vi "encoder_test_3mode.vi"() -> ()   [LabVIEW 2014]
uses:
  <vilib>/rvi/FXPMathLib/FxpSinAndCos/subVIs/nifxpmath_SinAndCos_SimConfig.ctl
  <vilib>/rvi/Emulation/niFpgaGetClockAttributes.vi
  <vilib>/rvi/Emulation/niFpgaSctlEmulationGetInTimedLoop.vi
  <vilib>/rvi/Emulation/niFpgaEmulationReportErrorSimple.vi
  <vilib>/rvi/eio/common/nirviEmuTemplateMethod_errors.vi
  <vilib>/rvi/Emulation/niFpgaProcessEmulError.vi
  <vilib>/rvi/Emulation/niFpgaCriticalErrorInLSC.vi
  <vilib>/rvi/FXPMathLib/FxpSinAndCos/simVIs/DllFxpSinAndCosTemp_sub.vi
  <vilib>/rvi/interface/RandomDataEmulation/nirviRandomDataMultiElementFPGAFIFO.vi
  <instcachedir>/0/nirviRandomDataMultiElementFPGAFIFO_AD0CFC12EF974623A9C2E4184BC062B2.lvgen/nirviRandomDataMultiElementFPGAFIFO_AD0CFC12EF974623A9C2E4184BC062B2_023.vi
  <vilib>/rvi/interface/RandomDataEmulation/niFpgaRandomDataHandleErrors.vi
  <vilib>/eio/EIONode/EIONode.xnode
  <vilib>/rvi/FXPMathLib/FxpMul/XNode/nifxpmath_Multiplier.xnode
  <vilib>/rvi/FXPMathLib/FxpSinAndCos/XNode/nifxpmath_SinAndCos.xnode
  <vilib>/rvi/Analysis/measure/butterworth/XNode/niFpgaButterworthFilter.xnode
  <vilib>/rvi/FXPMathLib/FxpSub/XNode/nifxpmath_Sub.xnode
  <vilib>/rvi/FXPMathLib/FxpAdd/XNode/nifxpmath_Add.xnode
  <vilib>/rvi/DataTransferAndStorage/Container/XNode/niFpgaContainer.xnode
  <vilib>/rvi/interface/RandomDataEmulation/nirviRandomDataFpgaMultiElementTemplate.vi
  <vilib>/rvi/FXPMathLib/sim/FxpSim.dll
panel:
  out "omega (M_avg)":fxp<+/-,64,35>
  out "D_d (M_avg)":fxp<+/-,64,32>
  in  "D_d_M_avg_Tc (uSec)":u32
  out "omega (M)":fxp<+/-,64,30>
  out "D_d (M)":fxp<+/-,64,27>
  in  "D_d_M_Tc (uSec)":u32 format="%#_6f"
  out "D_d (T)":fxp<+/-,46,10>
  out "omega(T)":fxp<+/-,20,9>
  in  "Velocity Estimation":i16(ring) items=["M_avg method", "M method", "T method"]
  out "Dr_ramp":fxp<+/-,64,30>
  out "Dr_slope":fxp<+/-,33,17>
  in  "Dr_time":fxp<+/-,16,11>
  out "Dr_sin":fxp<+/-,28,11>
  out "Dr_sin_d":fxp<+/-,64,16>
  out "Dr_sin_dd":fxp<+/-,64,25>
  out "Sin omega":fxp<+/-,41,8>
  in  "Sin offset":fxp<+/-,27,10>
  in  "Sin magnitude":fxp<+/-,11,8>
  in  "Sin wave frequency (Hz)":fxp<+/-,21,5>
  out "Time now (s)":fxp<+,52,14>
  out "Dr":fxp<+/-,64,31>
  in  "Dr_end":fxp<+/-,16,11>
  in  "Command type":i16(ring) items=["Step", "Ramp", "Sine"]
  out "D_i":fxp<+/-,34,18>
  in  "D_tolorence":fxp<+/-,14,3>
  in  "Ki":fxp<+/-,20,6>
  out "D_error":fxp<+/-,24,11>
  in  "Direction":bool
  out "Fmr_PD":fxp<+/-,64,31>
  in  "Kd":fxp<+/-,20,8>
  in  "Kp":fxp<+/-,20,12>
  in  "scaled coefficients_D_dd":i32[](array[numeric])=[780119100, 146811362]
  out "D_dd":fxp<+/-,36,29>
  in  "Ini coe.":bool
  out "va":fxp<+/-,38,8>
  out "vb":fxp<+/-,38,8>
  in  "stop motor":bool
  out "vq_F":fxp<+/-,20,5> format="%.57g"
  out "vd_F":fxp<+/-,20,5>
  out "D_d (mm/s)":fxp<+/-,32,12>
  out "mt":u32
  out "omega (rad/s)":fxp<+/-,32,18>
  in  "mt0":u32
  out "D(mm)":fxp<+/-,22,7>
  out "rad(NrTheta)":fxp<+/-,33,18>
  out "Encoder Position":i32
  in  "Encoder Reset":bool
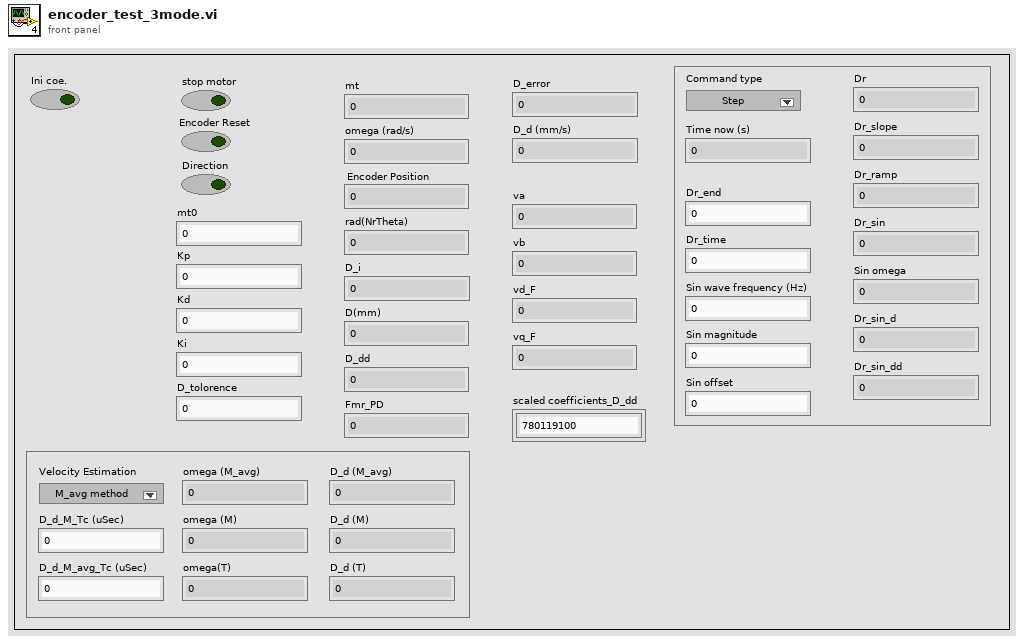
[diagram p1: front panel]
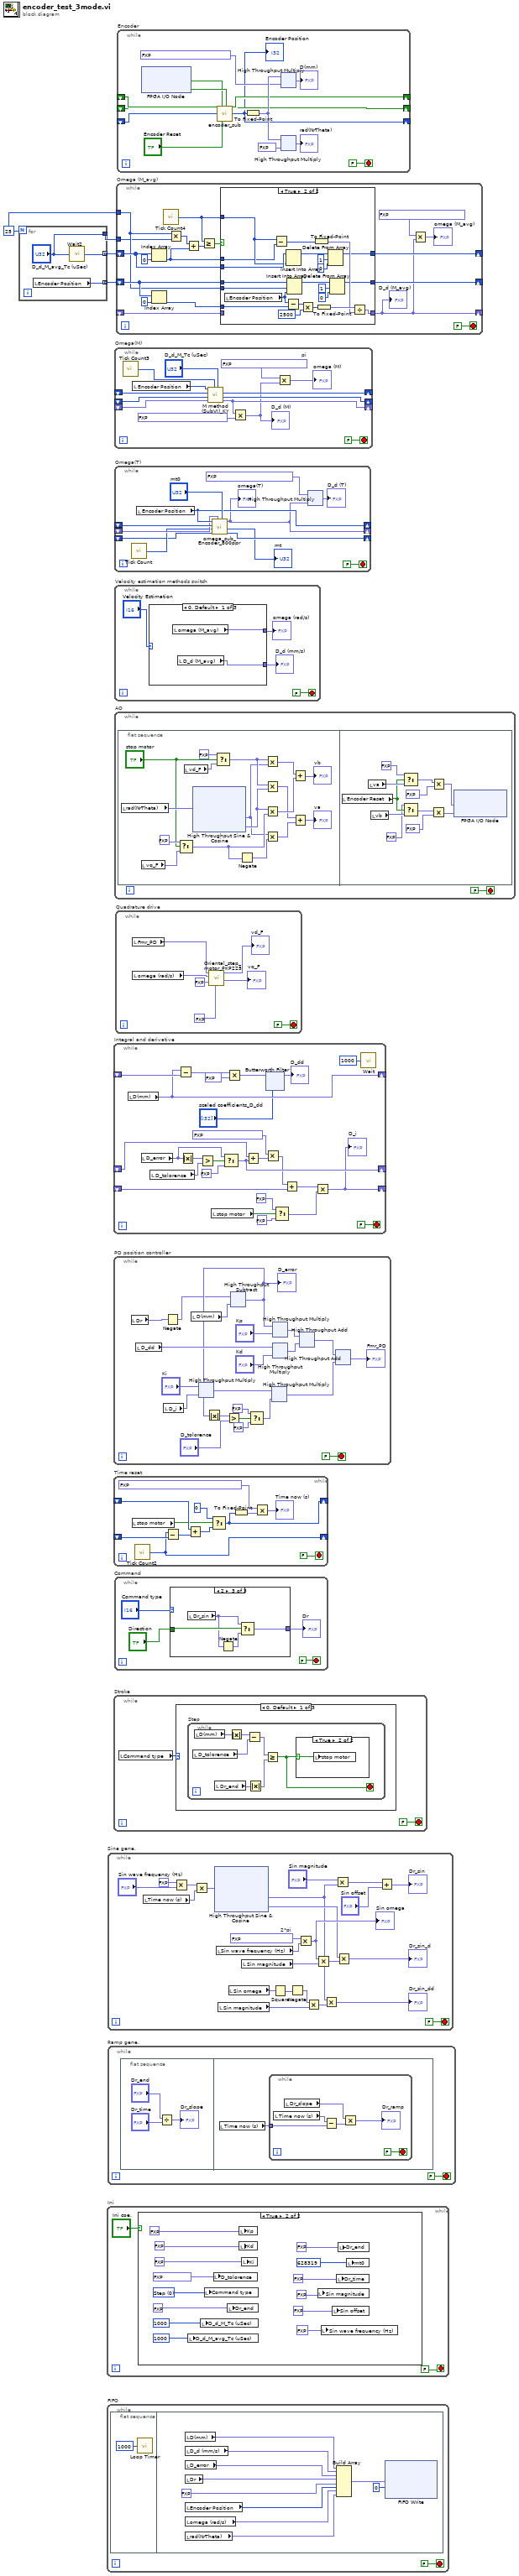
[diagram p0: block diagram]
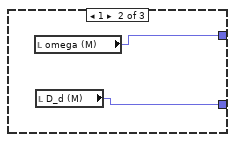
[diagram p3: hidden frame]
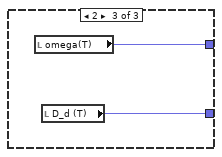
[diagram p4: hidden frame]
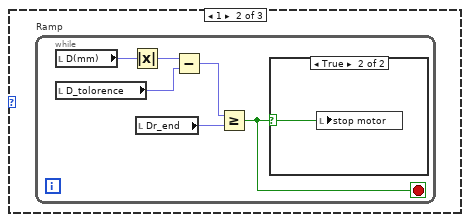
[diagram p6: hidden frame]
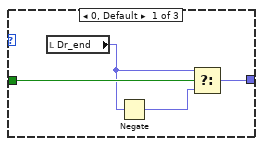
[diagram p9: hidden frame]
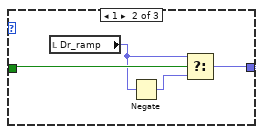
[diagram p10: hidden frame]
diagram:
  w4 = 25
  n1 = for {
    N: w4 -> [_]
    tunnel: ["D_d_M_avg_Tc (uSec)"] -> w1
    tunnel: [w6] -> w3 mode=indexing
    tunnel: [w5] -> w2 mode=indexing
    n2 = local read "Encoder Position"() -> (w5:i32)
    n3 = call "Wait2"("Count(uSec)"="D_d_M_avg_Tc (uSec)") -> ("Tick Count(uSec)"=w6:u32)
  }
  n4 = while "Ini" {
    stop <- FALSE stop-if-true
    n5 = case shown="True" "Ini coe." {
      frame False {
      }
      frame True {
        w17 = i16 0 items=["Step", "Ramp", "Sine"] ("Command type")
        n6 = local write "D_d_M_avg_Tc (uSec)"(u32 1000 ("D_d_M_avg_Tc (uSec)")) -> ()
        n7 = local write "D_d_M_Tc (uSec)"(u32 1000 ("D_d_M_Tc (uSec)")) -> ()
        n8 = local write "Command type"(w17) -> ()
        n9 = local write "D_tolorence"(fxp<+/-,14,3> 0.009765625 ("D_tolorence")) -> ()
        n10 = local write "Dr_end"(fxp<+/-,16,11> 20.0 ("Dr_end")) -> ()
        n11 = local write "Kp"(fxp<+/-,20,12> 10.0 ("Kp")) -> ()
        n12 = local write "Kd"(fxp<+/-,20,8> 2.0 ("Kd")) -> ()
        n13 = local write "Ki"(fxp<+/-,20,6> 8.0 ("D_i")) -> ()
        n14 = local write "Sin magnitude"(fxp<+/-,11,8> 20.0 ("Sin magnitude")) -> ()
        n15 = local write "Sin wave frequency (Hz)"(fxp<+/-,21,5> 0.5 ("Sin wave frequency (Hz)")) -> ()
        n16 = local write "Sin offset"(fxp<+/-,27,10> 0.0 ("Sin offset")) -> ()
        n17 = local write "Dr_time"(fxp<+/-,16,11> 5.0 ("Dr_time")) -> ()
        n18 = local write "Dr_end"(fxp<+/-,11,7> 20.0 ("Fmr")) -> ()
        n19 = local write "mt0"(u32 628319 ("mt0")) -> ()
      }
    }
  }
  n20 = while "FIFO" {
    stop <- FALSE stop-if-true
    n21 = flat-sequence {
      frame #0 {
        n22 = call "Loop Timer"("Count(uSec)"=u32 1000) -> ()  [unwired: 1 out]
      }
      frame #1 {
        n23 = local read "D(mm)"() -> (w33:fxp<+/-,22,7>)
        n24 = local read "D_d (mm/s)"() -> (w32:fxp<+/-,32,12>)
        n25 = local read "D_error"() -> (w31:fxp<+/-,24,11>)
        n26 = local read "Dr"() -> (w30:fxp<+/-,64,31>)
        n27 = local read "Encoder Position"() -> (w29:i32)
        n28 = local read "omega (rad/s)"() -> (w28:fxp<+/-,32,18>)
        n29 = local read "rad(NrTheta)"() -> (w27:fxp<+/-,33,18>)
        n30 = Build Array(w33, w32, w31, w30, fxp<+/-,64,32> 0.0 ("element"), w29, w28, w27) -> (w34:fxp<+/-,64,32>[])
        n31 = xnode ("FIFO Write")("Element"=w34, "Timeout"=0) -> ()  [unwired: 1 in, 2 out]
      }
    }
  }
  n32 = while "Sine gene." {
    stop <- FALSE stop-if-true
    w53 = fxp<+,20,3> 6.2831878662109375  # 2*pi
    n33 = local read "Time now (s)"() -> (w56:fxp<+,52,14>)
    n34 = Multiply(x=fxp<+,1,2> 2.0, y="Sin wave frequency (Hz)") -> (x*y=w57:fxp<+/-,21,6>)
    n35 = Multiply(x=w57, y=w56) -> (x*y=w37:fxp<+/-,64,20>)
    n36 = xnode "High Throughput Sine & Cosine"("x (pi)"=w37) -> ("sin(x)"=w41:fxp<+/-,16,2>, "cos(x)"=w48:fxp<+/-,16,2>)
    n37 = local read "Sin wave frequency (Hz)"() -> (w52:fxp<+/-,21,5>)
    n38 = local read "Sin magnitude"() -> (w43:fxp<+/-,11,8>)
    n39 = local read "Sin omega"() -> (w44:fxp<+/-,41,8>)
    n40 = local read "Sin magnitude"() -> (w47:fxp<+/-,11,8>)
    n41 = Square(x=w44) -> (x^2=w45:fxp<+,64,14>)
    n42 = Negate(x=w45) -> (-x=w42:fxp<+/-,64,15>)
    n43 = Multiply(x=w53, y=w52) -> (x*y=w49:fxp<+/-,41,8>)
    "Sin omega" <- w49
    n44 = Multiply(x=w42, y=w43) -> (x*y=w46:fxp<+/-,64,23>)
    n45 = Multiply(x=w49, y=w47) -> (x*y=w54:fxp<+/-,51,15>)
    n46 = Multiply(x=w41, y=w46) -> (x*y=→"Dr_sin_dd":fxp<+/-,64,25>)
    n47 = Multiply(x="Sin magnitude", y=w41) -> (x*y=w55:fxp<+/-,27,10>)
    n48 = Multiply(x=w48, y=w54) -> (x*y=→"Dr_sin_d":fxp<+/-,64,16>)
    n49 = Add(x=w55, y="Sin offset") -> (x+y=→"Dr_sin":fxp<+/-,28,11>)
  }
  n50 = while "Ramp gene." {
    stop <- FALSE stop-if-true
    n51 = flat-sequence {
      frame #0 {
        n52 = Divide(x="Dr_end", y="Dr_time") -> (x/y=→"Dr_slope":fxp<+/-,33,17>)
      }
      frame #1 {
        n53 = local read "Time now (s)"() -> (w94:fxp<+,52,14>)
        n54 = while {
          tunnel: w94 -> [w100]
          stop <- FALSE stop-if-true
          n55 = local read "Time now (s)"() -> (w97:fxp<+,52,14>)
          n56 = local read "Dr_slope"() -> (w98:fxp<+/-,33,17>)
          n57 = Subtract(x=w97, y=w100) -> (x-y=w99:fxp<+/-,53,15>)
          n58 = Multiply(x=w98, y=w99) -> (x*y=→"Dr_ramp":fxp<+/-,64,30>)
        }
      }
    }
  }
  n59 = while "Integral and derivative" {
    shift-right: [w121] -> _
    shift-left: _ -> [w125]
    shift-right: [w111] -> _
    shift-left: _ -> [w112]
    shift-right: [w101] -> _
    shift-left: _ -> [w105]
    stop <- FALSE stop-if-true
    n60 = local read "D(mm)"() -> (w121:fxp<+/-,22,7>)
    n61 = local read "D_error"() -> (w113:fxp<+/-,24,11>)
    n62 = local read "D_tolorence"() -> (w116:fxp<+/-,14,3>)
    n63 = Subtract(x=w121, y=w125) -> (x-y=w124:fxp<+/-,23,8>)
    n64 = Absolute Value(x=w113) -> (abs(x)=w117:fxp<+,24,11>)
    n65 = Greater?(x=w117, y=w116) -> (0:w115:bool)
    n66 = local read "stop motor"() -> (w108:bool)
    n67 = Select(t=w113, s=w115, f=fxp<+,24,11> 0.0) -> (s? t:f=w111:fxp<+/-,25,12>)
    n68 = Multiply(x=w124, y=fxp<+/-,33,13> 1000.0) -> (x*y=w122:fxp<+/-,55,20>)
    n69 = Add(x=w112, y=w111) -> (x+y=w110:fxp<+/-,26,13>)
    n70 = Multiply(x=fxp<+/-,30,12> 0.000499725341796875, y=w110) -> (x*y=w104:fxp<+/-,55,24>)
    n71 = xnode "Butterworth Filter"("input data"=w122, "scaled coefficients"="scaled coefficients_D_dd") -> ("output data"=→"D_dd":fxp<+/-,36,24>)  [unwired: 1 in]
    n72 = Select(t=fxp<+,1,1> 0.0, s=w108, f=fxp<+,1,1> 1.0) -> (s? t:f=w102:fxp<+,1,1>)
    n73 = Add(x=w104, y=w105) -> (x+y=w103:fxp<+/-,32,16>)
    n74 = Multiply(x=w103, y=w102) -> (x*y=w101:fxp<+/-,32,16>)
    "D_i" <- w101
    n75 = call "Wait"("Count(uSec)"=u32 1000) -> ()  [unwired: 1 out]
  }
  n76 = while "PD position controller" {
    stop <- FALSE stop-if-true
    n77 = local read "Dr"() -> (w136:fxp<+/-,64,31>)
    n78 = local read "D_dd"() -> (w152:fxp<+/-,36,29>)
    n79 = local read "D_i"() -> (w147:fxp<+/-,34,18>)
    n80 = Negate(x=w136) -> (-x=w135:fxp<+/-,64,32>)
    n81 = local read "D(mm)"() -> (w156:fxp<+/-,22,7>)
    n82 = xnode ("High Throughput Multiply")("x"="Ki", "y"=w147) -> ("x*y"=w141:fxp<+/-,54,24>)
    n83 = xnode "High Throughput Subtract"("x"=w135, "y"=w156) -> ("x-y"=w145:fxp<+/-,64,33>)
    "D_error" <- w145
    n84 = Absolute Value(x=w145) -> (abs(x)=w146:fxp<+,64,33>)
    n85 = Greater?(x=w146, y="D_tolorence") -> (0:w144:bool)
    n86 = Select(t=fxp<+,10,2> 1.0, s=w144, f=fxp<+,10,2> 0.0) -> (s? t:f=w140:fxp<+,10,2>)
    n87 = xnode ("High Throughput Multiply")("x"=w141, "y"=w140) -> ("x*y"=w137:fxp<+/-,64,26>)
    n88 = xnode ("High Throughput Multiply")("x"=w145, "y"="Kp") -> ("x*y"=w154:fxp<+/-,64,45>)
    n89 = xnode ("High Throughput Multiply")("x"=w152, "y"="Kd") -> ("x*y"=w153:fxp<+/-,56,37>)
    n90 = xnode ("High Throughput Add")("x"=w154, "y"=w153) -> ("x+y"=w138:fxp<+/-,64,46>)
    n91 = xnode ("High Throughput Add")("x"=w138, "y"=w137) -> ("x+y"=→"Fmr_PD":fxp<+/-,64,47>)
  }
  n92 = while "Time reset" {
    shift-right: [w160] -> _
    shift-left: _ -> [w167]
    shift-right: [w162] -> _
    shift-left: _ -> [w163]
    stop <- FALSE stop-if-true
    n93 = local read "stop motor"() -> (w165:bool)
    n94 = call "Tick Count2"() -> ("Tick Count(uSec)"=w162:u32)
    n95 = Subtract(x=w162, y=w163) -> (x-y=w168:u32)
    n96 = Add(x=w167, y=w168) -> (x+y=w166:u32)
    n97 = Select(t=u32 0, s=w165, f=w166) -> (s? t:f=w160:u32)
    n98 = To Fixed-Point(number=w160) -> (fixed-point=w159:fxp<+,32,32>)  [unwired: 1 in]
    n99 = Multiply(x=fxp<+,20,-18> 1.0000003385357559e-06, y=w159) -> (x*y=→"Time now (s)":fxp<+,52,14>)
  }
  n100 = while "Stroke" {
    stop <- FALSE stop-if-true
    n101 = local read "Command type"() -> (w170:i16)
    n102 = case shown="0, Default" w170 {
      frame 0, Default {
        n103 = while "Step" {
          stop <- w171 stop-if-true
          n104 = local read "D_tolorence"() -> (w173:fxp<+/-,14,3>)
          n105 = local read "D(mm)"() -> (w175:fxp<+/-,22,7>)
          n106 = local read "Dr_end"() -> (w177:fxp<+/-,16,11>)
          n107 = Absolute Value(x=w175) -> (abs(x)=w174:fxp<+,22,7>)
          n108 = Subtract(x=w174, y=w173) -> (x-y=w172:fxp<+/-,23,8>)
          n109 = Absolute Value(x=w177) -> (abs(x)=w176:fxp<+,16,11>)
          n110 = Greater Or Equal?(x=w172, y=w176) -> (x >= y?=w171:bool)
          n111 = case shown="True" w171 {
            selector: w171 -> [_ w178]
            frame False {
            }
            frame True {
              n112 = local write "stop motor"(w178) -> ()
            }
          }
        }
      }
      frame 1 {
        n113 = while "Ramp" {
          stop <- w179 stop-if-true
          n114 = local read "D(mm)"() -> (w181:fxp<+/-,22,7>)
          n115 = local read "D_tolorence"() -> (w183:fxp<+/-,14,3>)
          n116 = Absolute Value(x=w181) -> (abs(x)=w182:fxp<+,22,7>)
          n117 = local read "Dr_end"() -> (w180:fxp<+/-,16,11>)
          n118 = Subtract(x=w182, y=w183) -> (x-y=w184:fxp<+/-,23,8>)
          n119 = Greater Or Equal?(x=w184, y=w180) -> (x >= y?=w179:bool)
          n120 = case shown="True" w179 {
            selector: w179 -> [_ w185]
            frame False {
            }
            frame True {
              n121 = local write "stop motor"(w185) -> ()
            }
          }
        }
      }
      frame 2 {
      }
    }
  }
  n122 = while "Command" {
    stop <- FALSE stop-if-true
    n123 = case shown="2" "Command type" {
      tunnel: [w190 w194 w198] -> w188
      tunnel: "Direction" -> [w193 w197 w201]
      frame 0, Default {
        n124 = local read "Dr_end"() -> (w192:fxp<+/-,16,11>)
        n125 = Negate(x=w192) -> (-x=w191:fxp<+/-,17,12>)
        n126 = Select(t=w192, s=w193, f=w191) -> (s? t:f=w190:fxp<+/-,17,12>)
      }
      frame 1 {
        n127 = local read "Dr_ramp"() -> (w195:fxp<+/-,64,30>)
        n128 = Negate(x=w195) -> (-x=w196:fxp<+/-,64,31>)
        n129 = Select(t=w195, s=w197, f=w196) -> (s? t:f=w194:fxp<+/-,64,31>)
      }
      frame 2 {
        n130 = local read "Dr_sin"() -> (w199:fxp<+/-,28,11>)
        n131 = Negate(x=w199) -> (-x=w200:fxp<+/-,27,10>)
        n132 = Select(t=w199, s=w201, f=w200) -> (s? t:f=w198:fxp<+/-,28,11>)
      }
    }
    "Dr" <- w188
  }
  n133 = while "Omega(M)" {
    shift-right: [w213] -> _
    shift-left: _ -> [w214]
    shift-right: [w209] -> _
    shift-left: _ -> [w210]
    shift-right: [w207] -> _
    shift-left: _ -> [w208]
    stop <- FALSE stop-if-true
    w204 = fxp<+/-,27,3> 3.1415926218032837  # pi
    n134 = call "Tick Count3"() -> ("Tick Count(mSec)"=w212:u32)
    n135 = local read "Encoder Position"() -> (w215:i32)
    n136 = call "M method (SubVI)_KY.vi"("Tc (mSec)"="D_d_M_Tc (uSec)", "Tick Count (mSec)"=w212, "Encoder velocity_pre (pulse/s)"=w208, "Shift Register in 2"=w210, "Shift Register in 1"=w214, "Encoder pulses"=w215) -> ("Encoder velocity (pulse/s)"=w207:fxp<+/-,64,32>, "Shift Register out 2"=w209:i32, "Shift Register out 1"=w213:u32)  [unwired: 3 in]
    n137 = Multiply(x=w207, y=fxp<+/-,20,-5> 0.002499997615814209) -> (x*y=w205:fxp<+/-,64,27>)
    "D_d (M)" <- w205
    n138 = Multiply(x=w204, y=w205) -> (x*y=→"omega (M)":fxp<+/-,64,30>)
  }
  n139 = while "Omega(T)" {
    shift-right: [w225] -> _
    shift-left: _ -> [w226]
    shift-right: [w218] -> _
    shift-left: _ -> [w224]
    shift-right: [w221] -> _
    shift-left: _ -> [w222]
    stop <- FALSE stop-if-true
    n140 = call "Tick Count"() -> ("Tick Count(Ticks)"=w223:u32)
    n141 = local read "Encoder Position"() -> (w225:i32)
    n142 = call "omega_sub_Encoder_800ppr.vi"("mt0"="mt0", "omega_pre"=w224, "ticks_m_pre"=w222, "ticks"=w223, "count_pre"=w226, "count"=w225) -> ("ticks_m"=w221:u32, "mt"=→"mt":u32, "omega"=w218:fxp<+/-,20,9>)  [unwired: 3 in]
    "omega(T)" <- w218
    n143 = xnode ("High Throughput Multiply")("x"=fxp<+/-,26,1> 0.3183099031448364, "y"=w218) -> ("x*y"=→"D_d (T)":fxp<+/-,46,10>)
  }
  n144 = while "Velocity estimation methods switch" {
    stop <- FALSE stop-if-true
    n145 = case shown="0, Default" "Velocity Estimation" {
      tunnel: [w233 w235 w237] -> w230
      tunnel: [w232 w234 w236] -> w229
      frame 0, Default {
        n146 = local read "omega (M_avg)"() -> (w233:fxp<+/-,64,35>)
        n147 = local read "D_d (M_avg)"() -> (w232:fxp<+/-,64,32>)
      }
      frame 1 {
        n148 = local read "omega (M)"() -> (w235:fxp<+/-,64,30>)
        n149 = local read "D_d (M)"() -> (w234:fxp<+/-,64,27>)
      }
      frame 2 {
        n150 = local read "omega(T)"() -> (w237:fxp<+/-,20,9>)
        n151 = local read "D_d (T)"() -> (w236:fxp<+/-,46,10>)
      }
    }
    "D_d (mm/s)" <- w229
    "omega (rad/s)" <- w230
  }
  n152 = while "AO" {
    stop <- FALSE stop-if-true
    n153 = flat-sequence {
      frame #0 {
        n154 = local read "rad(NrTheta)"() -> (w254:fxp<+/-,33,18>)
        n155 = local read "vq_F"() -> (w252:fxp<+/-,20,5>)
        n156 = Select(t=fxp<+,20,5> 0.0, s="stop motor", f=w252) -> (s? t:f=w249:fxp<+/-,21,6>)
        n157 = local read "vd_F"() -> (w253:fxp<+/-,20,5>)
        n158 = xnode "High Throughput Sine & Cosine"("x (pi)"=w254) -> ("sin(x)"=w245:fxp<+/-,17,2>, "cos(x)"=w247:fxp<+/-,17,2>)
        n159 = Select(t=fxp<+,20,5> 0.0, s="stop motor", f=w253) -> (s? t:f=w246:fxp<+/-,21,6>)
        n160 = Negate(x=w249) -> (-x=w248:fxp<+/-,21,6>)
        n161 = Multiply(x=w246, y=w245) -> (x*y=w244:fxp<+/-,37,7>)
        n162 = Multiply(x=w246, y=w247) -> (x*y=w242:fxp<+/-,37,7>)
        n163 = Multiply(x=w247, y=w249) -> (x*y=w243:fxp<+/-,37,7>)
        n164 = Multiply(x=w245, y=w248) -> (x*y=w241:fxp<+/-,37,7>)
        n165 = Add(x=w244, y=w243) -> (x+y=→"vb":fxp<+/-,38,8>)
        n166 = Add(x=w242, y=w241) -> (x+y=→"va":fxp<+/-,38,8>)
      }
      frame #1 {
        n167 = local read "Encoder Reset"() -> (w288:bool)
        n168 = local read "va"() -> (w290:fxp<+/-,38,8>)
        n169 = local read "vb"() -> (w289:fxp<+/-,38,8>)
        n170 = Select(t=fxp<+/-,20,5> 5.0 ("y"), s=w288, f=w290) -> (s? t:f=w291:fxp<+/-,38,8>)
        n171 = Select(t=fxp<+/-,20,5> 0.0 ("y"), s=w288, f=w289) -> (s? t:f=w292:fxp<+/-,38,8>)
        n172 = Multiply(x=w292, y=fxp<+/-,20,5> -0.5) -> (x*y=w296:fxp<+/-,57,12>)
        n173 = Multiply(x=w291, y=fxp<+/-,20,5> -0.5) -> (x*y=w295:fxp<+/-,57,12>)
        n174 = xnode "FPGA I/O Node"("Mod8/AO0"=w295, "Mod8/AO1"=w296) -> ()  [unwired: 2 in, 2 out]
      }
    }
  }
  n175 = while "Quadrature drive" {
    stop <- FALSE stop-if-true
    n176 = local read "Fmr_PD"() -> (w297:fxp<+/-,64,31>)
    n177 = local read "omega (rad/s)"() -> (w299:fxp<+/-,32,18>)
    n178 = call "Oriental_step_motor_PKP225.vi"("F_Threshold"=fxp<+,12,12> 10.0, "dFmr"=fxp<+/-,25,15> 0.0, "omega"=w299, "Fmr"=w297) -> ("vq_F"=→"vq_F":fxp<+/-,20,5>, "vd_F"=→"vd_F":fxp<+/-,20,5>)  [unwired: 6 in]
  }
  n179 = while "Omega (M_avg)" {
    tunnel: w4 -> [w315]
    shift-right: [w308] -> _
    shift-left: w3 -> [w319]
    shift-right: [w307] -> _
    shift-left: _ -> [w310]
    shift-right: [w309] -> _
    shift-left: w2 -> [w318]
    tunnel: w1 -> [w312]
    stop <- FALSE stop-if-true
    n180 = Index Array(array=w319, index=0) -> (element=w313:u32)
    n181 = Index Array(array=w318, index=0) -> (element=w314:i32)
    n182 = call "Tick Count4"() -> ("Tick Count(uSec)"=w316:u32)
    n183 = Multiply(x=w315, y=w312) -> (x*y=w320:u32)
    n184 = Add(x=w320, y=w313) -> (x+y=w317:u32)
    n185 = Greater Or Equal?(x=w316, y=w317) -> (x >= y?=w311:bool)
    n186 = case shown="True" w311 {
      tunnel: w319 -> [w325 w342]
      tunnel: w318 -> [w324 w341]
      tunnel: w316 -> [_ w334]
      tunnel: w315 -> [_ w340]
      tunnel: w314 -> [_ w338]
      tunnel: w313 -> [_ w333]
      tunnel: w310 -> [w323 _]
      tunnel: [w324 w328] -> w309
      tunnel: [w325 w327] -> w308
      tunnel: [w323 w326] -> w307
      frame False {
      }
      frame True {
        n187 = local read "Encoder Position"() -> (w339:i32)
        n188 = Subtract(x=w334, y=w333) -> (x-y=w331:u32)
        n189 = Insert Into Array(array=w342, new element=w334) -> (w343:u32[])  [unwired: 1 in]
        n190 = Subtract(x=w339, y=w338) -> (x-y=w337:i32)
        n191 = Insert Into Array(array=w341, index=w340, new element=w339) -> (w344:i32[])
        n192 = Multiply(x=w337, y=2500) -> (x*y=w335:i32)
        n193 = To Fixed-Point(number=w331) -> (fixed-point=w329:fxp<+,32,32>)  [unwired: 1 in]
        n194 = To Fixed-Point(number=w335) -> (fixed-point=w330:fxp<+/-,32,32>)  [unwired: 1 in]
        n195 = Delete From Array(array=w343, length=1, index=0) -> (array with subset deleted=w327:u32[])  [unwired: 1 out]
        n196 = Delete From Array(array=w344, length=1, index=0) -> (array with subset deleted=w328:i32[])  [unwired: 1 out]
        n197 = Divide(x=w330, y=w329) -> (x/y=w326:fxp<+/-,64,32>)
      }
    }
    "D_d (M_avg)" <- w307
    n198 = Multiply(x=fxp<+/-,27,3> 3.1415926218032837, y=w307) -> (x*y=→"omega (M_avg)":fxp<+/-,64,35>)
  }
  n199 = while "Encoder" {
    shift-right: [w354] -> _
    shift-left: _ -> [w356]
    shift-right: [w353] -> _
    shift-left: _ -> [w355]
    shift-right: [w351] -> _
    shift-left: _ -> [w352]
    stop <- FALSE stop-if-true
    n200 = xnode "FPGA I/O Node"() -> ("Mod4/DI3"=w361:bool, "Mod4/DI4"=w362:bool)  [unwired: 2 in, 2 out]
    n201 = call "encoder_sub.vi"("A_pre"=w356, "B_pre"=w355, "Encoder Position_pre"=w352, "A input"=w361, "Encoder Position Reset"="Encoder Reset", "B input"=w362) -> ("A"=w354:bool, "B"=w353:bool, "Encoder Position (Counts)"=w351:i32)  [unwired: 19 in]
    "Encoder Position" <- w351
    n202 = To Fixed-Point(number=w351) -> (fixed-point=w359:fxp<+/-,32,32>)  [unwired: 1 in]
    n203 = xnode ("High Throughput Multiply")("x"=w359, "y"=fxp<+/-,24,0> 0.002499997615814209) -> ("x*y"=→"D(mm)":fxp<+/-,56,32>)
    n204 = xnode ("High Throughput Multiply")("x"=w359, "y"=fxp<+/-,24,0> 0.125) -> ("x*y"=→"rad(NrTheta)":fxp<+/-,56,32>)
  }
